vi "Get Children.vi"(8 "error in (no error)":errorcluster, 9 "tag index":i32, 10 "child name (\"\": all children)":string, 11 "xml structure in":T1) -> (0 "error out":errorcluster, 1 "child indices":i32[](array[numeric]), 2 "child names":string[](array[string]), 3 "xml structure out":T1)   [LabVIEW 2013]
uses:
  XML Structure - Cluster.ctl
  XML Tag Type - Enum.ctl
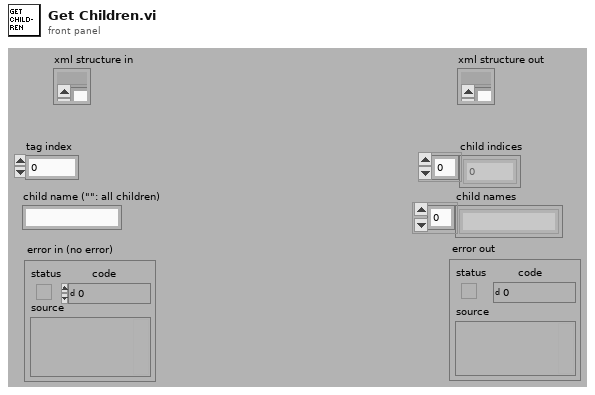
[diagram p1: front panel]
types:
  T1 = typedef "XML Structure - Cluster.ctl" = cluster{"tags":string[], "tag names":string[], "tag type":T2[], "offset":i32[], "close tag index":i32[], "xml":string, "Children":cluster{"children":i32[]}[], "parent index":i32[]}
  T2 = typedef "XML Tag Type - Enum.ctl" = enum16{"start tag", "empty tag", "end tag"}
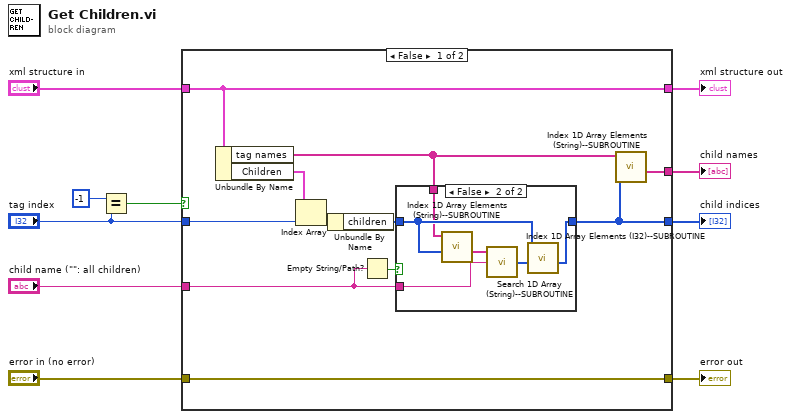
[diagram p0: block diagram]
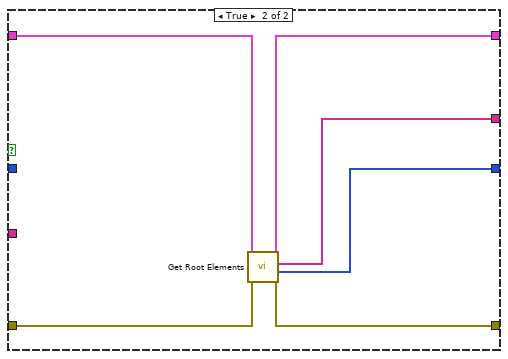
[diagram p3: hidden frame]
diagram:
  n1 = Equal?(x=-1, y="tag index") -> (x = y?=w2:bool)
  n2 = case shown="False" w2 {
    tunnel: "xml structure in" -> [w11 w29]
    tunnel: "tag index" -> [w21 _]
    tunnel: [w17 w32] -> w9
    tunnel: [w15 w31] -> w8
    tunnel: "child name (\"\": all children)" -> [w13 _]
    tunnel: [w12 w33] -> w6
    tunnel: "error in (no error)" -> [w12 w34]
    tunnel: [w11 w30] -> w1
    frame False {
      n3 = Unbundle By Name(w11) -> ("tag names"=w16:string[], "Children"=w20:cluster{"children":i32[]}[])
      n4 = Index Array(array=w20, index=w21) -> (element=w19:cluster{"children":i32[]})
      n5 = Unbundle By Name(w19) -> ("children"=w18:i32[])
      n6 = Empty String/Path?(string/path=w13) -> (empty?=w14:bool)
      n7 = case shown="False" w14 {
        tunnel: w13 -> [_ w28]
        tunnel: w18 -> [w22 w25]
        tunnel: [w22 w24] -> w17
        tunnel: w16 -> [_ w23]
        frame True {
        }
        frame False {
          n8 = call "Index 1D Array Elements (String)--SUBROUTINE.vi"("indices"=w25, "array"=w23) -> ("elements"=w27:string[])  [unwired: 9 in]
          n9 = call "Search 1D Array (String)--SUBROUTINE.vi"("Array"=w27, "Element Data"=w28) -> ("Indices of Elements"=w26:i32[])  [unwired: 7 in]
          n10 = call "Index 1D Array Elements (I32)--SUBROUTINE.vi"("indices"=w26, "array"=w25) -> ("elements"=w24:i32[])  [unwired: 9 in]
        }
      }
      n11 = call "Index 1D Array Elements (String)--SUBROUTINE.vi"("indices"=w17, "array"=w16) -> ("elements"=w15:string[])  [unwired: 9 in]
    }
    frame True {
      n12 = call "Get Root Elements.vi"("error in (no error)"=w34, "xml structure in"=w29) -> ("error out"=w33:errorcluster, "tag indices"=w32:i32[], "tag names"=w31:string[], "xml structure out"=w30:T1)  [unwired: 6 in]
    }
  }
  "xml structure out" <- w1
  "child indices" <- w9
  "error out" <- w6
  "child names" <- w8
